vi "arqui1.vi"() -> ()   [LabVIEW 2026]
uses:
  <vilib>/Utility/file.llb/Read Delimited Spreadsheet (DBL).vi
  <vilib>/Analysis/NI_AALPro.lvlib
panel:
  out "Array":dbl[](array[numeric])
  out "intercept":dbl
  out "slope":dbl
  out "XY Graph":T1(graph)
  out "y":dbl[](array[numeric])
  out "x":dbl[](array[numeric])
  out "all rows":dbl[][](array[numeric])
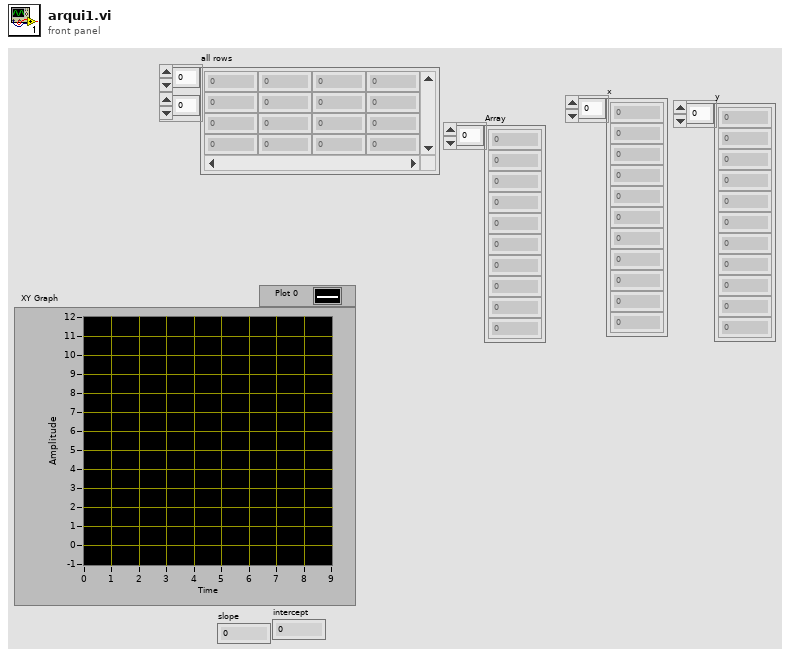
[diagram p1: front panel]
types:
  T1 = cluster{"all rows":dbl[], "Best Linear Fit":dbl[]}[]
  T2 = cluster{"all rows":dbl[], "Best Linear Fit":dbl[]}
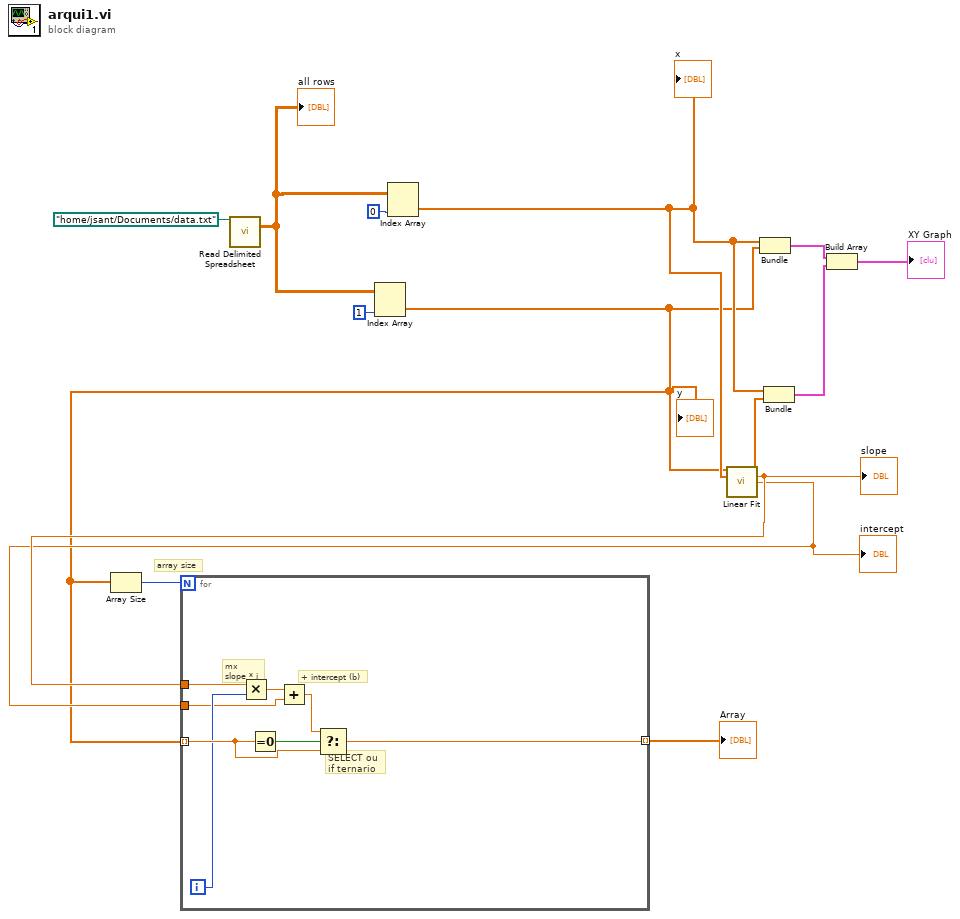
[diagram p0: block diagram]
diagram:
  # "array size"
  n1 = call-poly <vilib>:"Read Delimited Spreadsheet.vi"("file path (dialog if empty)"=path "/home/jsant/Documents/data.txt") -> ("all rows"=w12:dbl[][])  [unwired: 9 in, 5 out]
  "all rows" <- w12
  n2 = Index Array(array=w12, index (col)=1 ("disabled index (col)")) -> (element=w1:dbl[])  [unwired: 1 in]
  "y" <- w1
  n3 = Array Size(array=w1) -> (size(s)=w2:i32)
  n4 = Index Array(array=w12, index (col)=0 ("disabled index (col)")) -> (element=w9:dbl[])  [unwired: 1 in]
  "x" <- w9
  n5 = call <vilib>:"Linear Fit.vi"("Y"=w1, "X"=w9) -> ("Best Linear Fit"=w10:dbl[], "slope"=w4:dbl, "intercept"=w3:dbl)  [unwired: 9 in, 2 out]
  "slope" <- w4
  "intercept" <- w3
  n6 = for {
    N: w2 -> [_]
    tunnel: w1 -> [w21] mode=indexing
    tunnel: [w20] -> w5 mode=indexing
    tunnel: w4 -> [w19]
    tunnel: w3 -> [w17]
    i -> [w18]
    # "+ intercept (b)"
    # "mx\nslope * i"
    # "SELECT ou\nif ternario"
    n7 = Multiply(x=w19, y=w18) -> (x*y=w16:dbl)
    n8 = Equal To 0?(x=w21) -> (x = 0?=w22:bool)
    n9 = Add(x=w16, y=w17) -> (x+y=w15:dbl)
    n10 = Select(t=w15, s=w22, f=w21) -> (s? t:f=w20:dbl)
  }
  "Array" <- w5
  n11 = Bundle("all rows"=w9, "all rows"=w1) -> (w8:cluster{"all rows":dbl[], "all rows":dbl[]})  [unwired: 1 in]
  n12 = Bundle("all rows"=w9, "Best Linear Fit"=w10) -> (w7:T2)  [unwired: 1 in]
  n13 = Build Array(w8, w7) -> (→"XY Graph":T1)
